vi "ADCP通讯.vi"(6 "Slave ID":u8=1, 7 "STEP":enum16{"open", "read", "write", "close"}(ring)=enum."read", 8 "Error in":errorcluster caption="Error in (no error)", 9 "values":u16[](array[numeric]), 10 "quantity":u16, 11 "starting address":u16) -> (0 "error out":errorcluster, 2 "输出簇":T1, 3 "Registers":u16[](array[numeric]))   [LabVIEW 2016, in "ADCP.lvlib"]
uses:
  ADCP.lvlib
  <vilib>/Plasmionique/MB Master/MB_ADU/MB_ADU.lvclass/MB_ADU.ctl
  <vilib>/Plasmionique/MB Master/MB_ADU/Read RX Data.vi
  <vilib>/Plasmionique/MB Master/MB_ADU/Read RX Timestamp.vi
  <vilib>/Plasmionique/MB Master/MB_ADU/Read Slave ID.vi
  <vilib>/Plasmionique/MB Master/MB_ADU/Read TX Data.vi
  <vilib>/Plasmionique/MB Master/MB_ADU/Read TX Timestamp.vi
  <vilib>/Plasmionique/MB Master/MB_Master_Serial/MB_Master_Serial.lvclass
  C:/Program Files (x86)/National Instruments/LabVIEW 2016/vi.lib/Plasmionique/MB Master/MB_Master/MB_Master.lvclass
  <vilib>/Plasmionique/MB Master/MB_ADU/MB_ADU.lvclass
  <vilib>/Plasmionique/MB Master/MB_Master/MB_Master.lvclass
  <vilib>/Plasmionique/MB Master/MB Master.lvlib
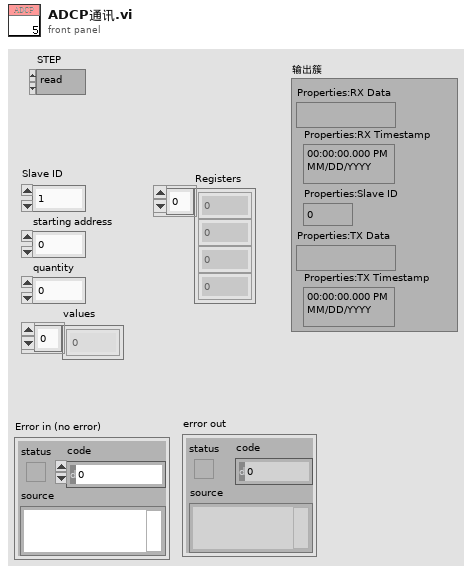
[diagram p1: front panel]
types:
  T1 = cluster{"Properties:RX Data":string, "Properties:RX Timestamp":timestamp, "Properties:Slave ID":u8, "Properties:TX Data":string, "Properties:TX Timestamp":timestamp}
  T2 = cluster{"baud rate (bps)":u32, "stop bits":u16, "parity":u16, "flow control":u16, "timeout":u32, "retries":i32}
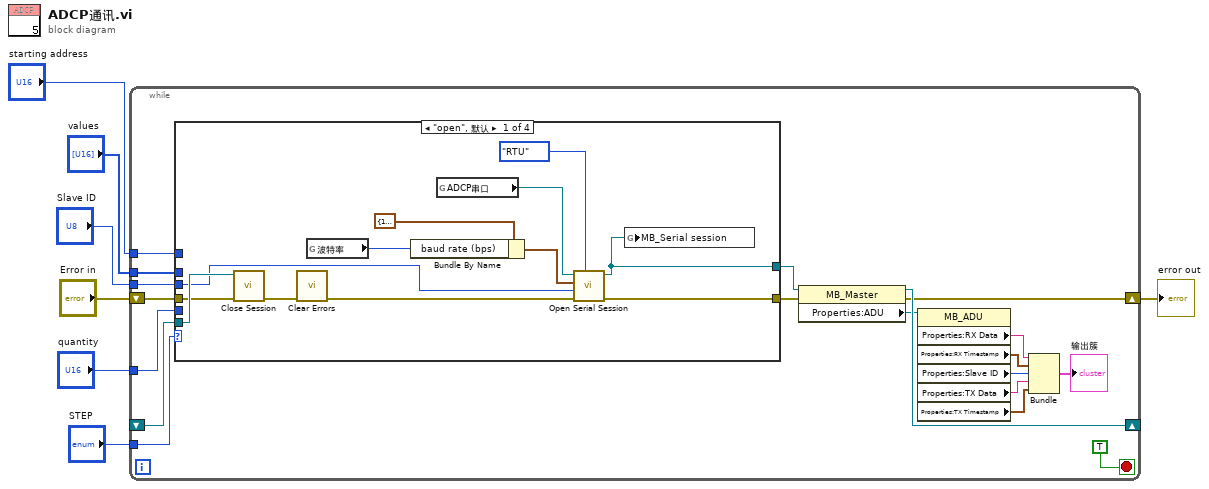
[diagram p0: block diagram]
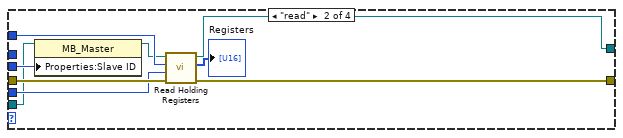
[diagram p2: hidden frame]
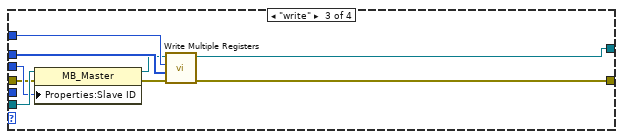
[diagram p3: hidden frame]
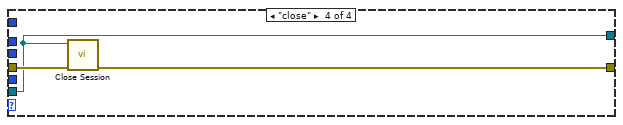
[diagram p4: hidden frame]
diagram:
  n1 = while {
    shift-right: [w20] -> _
    shift-left: _ -> [w26]
    shift-right: [w18] -> w6
    shift-left: "Error in" -> [w25]
    tunnel: "Slave ID" -> [w24]
    tunnel: "starting address" -> [w23]
    tunnel: "quantity" -> [w22]
    tunnel: "STEP" -> [w21]
    tunnel: "values" -> [w11]
    stop <- TRUE stop-if-true
    n2 = case shown="\"open\", 默认" w21 {
      tunnel: w26 -> [w36 w40 w52 w57]
      tunnel: w25 -> [w35 w47 w49 w59]
      tunnel: [w30 w46 w55 w57] -> w8
      tunnel: [w37 w45 w56 w58] -> w19
      tunnel: w24 -> [w29 w43 w51 _]
      tunnel: w23 -> [_ w42 w54 _]
      tunnel: w22 -> [_ w41 _ _]
      tunnel: w11 -> [_ _ w53 _]
      frame "open", Default {
        n3 = call-dynamic "Close Session.vi"("error in (no error)"=w35, "MB session in"=w36) -> ("error out"=w28:errorcluster)  [unwired: 9 in]
        n4 = call <vilib>:"Clear Errors.vi"("error in (no error)"=w28) -> ("error out"=w27:errorcluster)  [unwired: 5 in, 1 out]
        n5 = global read "ADCP全局变量.vi" "波特率"() -> (w32:u32)
        n6 = Bundle By Name(cluster=T2 {"baud rate (bps)"=115200, "stop bits"=10, "parity"=0, "flow control"=0, "timeout"=500, "retries"=1} ("Serial Config"), "baud rate (bps)"=w32) -> (w33:T2)
        n7 = global read "ADCP全局变量.vi" "ADCP串口"() -> (w31:refnum<visa-resource-name>)
        n8 = call <vilib>:"Open Serial Session.vi"("Mode (RTU)"=enum16{"RTU", "ASCII"}."RTU", "Error in"=w27, "Slave ID"=w29, "Serial Config"=w33, "VISA Resource"=w31) -> ("Error out"=w37:errorcluster, "MB_Serial session"=w30:refnum<class "MB_Master_Serial.lvclass">)  [unwired: 5 in]
        n9 = global write "ADCP全局变量.vi" "MB_Serial session"(w30) -> ()
      }
      frame "read" {
        n10 = property class="MB_Master"(reference=w40, "Properties:Slave ID"=w43) -> (reference out=w39:refnum<class "MB_Master.lvclass">)  [unwired: 1 in, 1 out]
        n11 = call <vilib>:"Read Holding Registers.vi"("error in (no error)"=w47, "quantity"=w41, "starting address"=w42, "MB session in"=w39) -> ("error out"=w45:errorcluster, "Registers"=→"Registers":u16[], "MB session out"=w46:refnum<class "MB_Master.lvclass">)  [unwired: 5 in]
      }
      frame "write" {
        n12 = property class="MB_Master"(reference=w52, error in=w49, "Properties:Slave ID"=w51) -> (reference out=w50:refnum<class "MB_Master.lvclass">, error out=w48:errorcluster)
        n13 = call <vilib>:"Write Multiple Registers.vi"("error in (no error)"=w48, "values"=w53, "starting address"=w54, "MB session in"=w50) -> ("error out"=w56:errorcluster, "MB session out"=w55:refnum<class "MB_Master.lvclass">)  [unwired: 6 in]
      }
      frame "close" {
        n14 = call-dynamic "Close Session.vi"("error in (no error)"=w59, "MB session in"=w57) -> ("error out"=w58:errorcluster)  [unwired: 9 in]
      }
    }
    n15 = property class="MB_Master"(reference=w8, error in=w19) -> (reference out=w20:refnum<class "MB_Master.lvclass">, error out=w18:errorcluster, "Properties:ADU"=w9:refnum<class "MB_ADU.lvclass">)
    n16 = property class="MB_ADU"(reference=w9) -> ("Properties:RX Data"=w17:string, "Properties:RX Timestamp"=w16:timestamp, "Properties:Slave ID"=w15:u8, "Properties:TX Data"=w14:string, "Properties:TX Timestamp"=w13:timestamp)  [unwired: 1 in, 2 out]
    n17 = Bundle("Properties:RX Data"=w17, "Properties:RX Timestamp"=w16, "Properties:Slave ID"=w15, "Properties:TX Data"=w14, "Properties:TX Timestamp"=w13) -> (→"输出簇":T1)  [unwired: 1 in]
  }
  "error out" <- w6
